vi "UV-VIS GetNumberPreAmpGainsSD.vi"(4 "error in (no error)":errorcluster, 7 "UV-VIS in":refnum<class "UV-VIS.lvclass">) -> (0 "error out":errorcluster, 1 "DLL error code":u32, 2 "number":i32, 3 "UV-VIS out":refnum<class "UV-VIS.lvclass">)   [LabVIEW 2015, in "UV-VIS.lvclass"]
doc: "Available in some systems are a number of pre amp gains that can be applied to the data as it is read out. This function gets the number of these gains available. The functions <B>GetPreAmpGain</B> and <B>SetPreAmpGain</B> can be used to specify which of these gains is to be used.\n\n<B>Parameter:</B>\nnumber - number of allowed pre amp gains\n\n<B>Error codes:</B>\nDRV_SUCCESS - Number of pre amp gains returned.\nDRV_NOT_INITIALIZED - System not initialized.\nDRV_ACQUIRING - Acquisition in progress."
uses:
  UV-VIS.lvclass
  Detector.lvclass/Detector.ctl
  Detector.lvclass
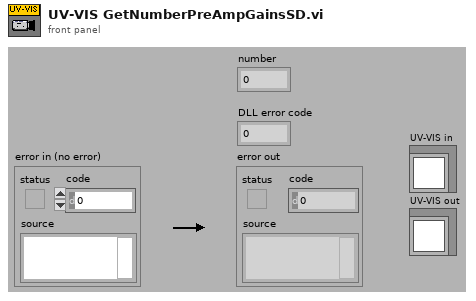
[diagram p1: front panel]
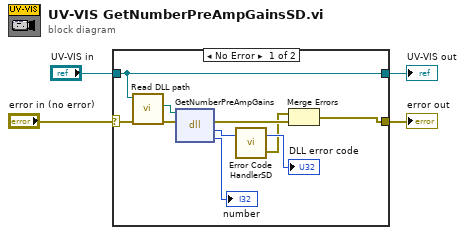
[diagram p0: block diagram]
diagram:
  n1 = case shown="No Error" "error in (no error)" {
    selector: "error in (no error)" -> [w11 w16]
    tunnel: [w5 w16] -> w3
    tunnel: [w10 w15] -> w2
    tunnel: "UV-VIS in" -> [w10 w15]
    frame No Error {
      n2 = call "Read DLL path.vi"("error in (no error)"=w11, "Detector in"=w10) -> ("error out"=w9:errorcluster, "DLL path"=w8:path)  [unwired: 7 in, 1 out]
      n3 = dll-call lib="S:/TRANCON/DLL/Atmcd32d.dll" fn="GetNumberPreAmpGains"(path in=w8, error in=w9) -> (error out=w7:errorcluster, "return type"=w14:u32, "number"=→"number":i32)  [unwired: 2 in, 1 out]
      n4 = call "Error Code HandlerSD.vi"("DLL error code"=w14) -> ("error out"=w6:errorcluster, "dup DLL error code"=→"DLL error code":u32)  [unwired: 1 in]
      n5 = Merge Errors(w6, w7) -> (w5:errorcluster)
    }
    frame Error {
    }
  }
  "error out" <- w3
  "UV-VIS out" <- w2
